vi "afd2matrix.vi"(0 "afd":cluster{i16[], i32[]}[](array[cluster])) -> (2 "Offset":dbl, 3 "Multiplier":dbl, 4 "Array":sgl[][](array[numeric]))   [LabVIEW 2010]
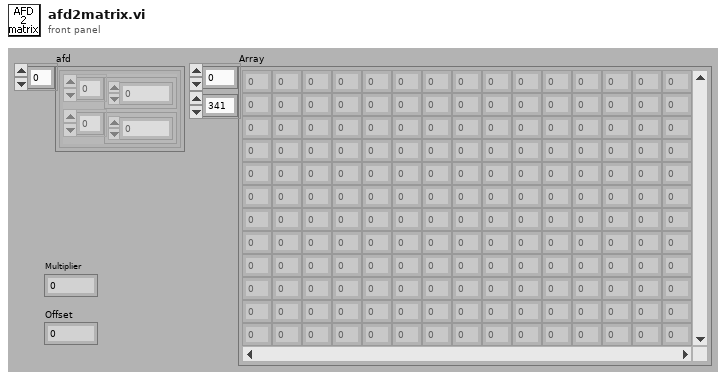
[diagram p1: front panel]
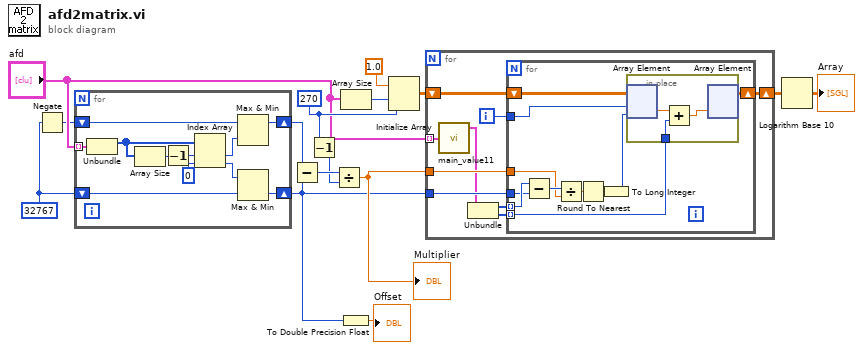
[diagram p0: block diagram]
diagram:
  w3 = i16 32767
  w8 = 270 ("dimension size")
  n1 = Negate(x=w3) -> (-x=w4:i16)
  n2 = for {
    tunnel: "afd" -> [w26] mode=indexing
    shift-right: [w17] -> w1
    shift-left: w3 -> [w16]
    shift-right: [w18] -> w2
    shift-left: w4 -> [w19]
    n3 = Unbundle(w26) -> (w22:i16[])  [unwired: 1 out]
    n4 = Array Size(array=w22) -> (size(s)=w24:i32)
    n5 = Decrement(x=w24) -> (x-1=w23:i32)
    n6 = Index Array(array=w22, index #1=w23, index #2=0 ("index")) -> (element #1=w20:i16, element #2=w21:i16)
    n7 = Max & Min(x=w19, y=w20) -> (max(x,y)=w18:i16)  [unwired: 1 out]
    n8 = Max & Min(x=w21, y=w16) -> (min(x,y)=w17:i16)  [unwired: 1 out]
  }
  n9 = Subtract(x=w2, y=w1) -> (x-y=w7:i16)
  n10 = Decrement(x=w8) -> (x-1=w6:i32)
  n11 = Divide(x=w7, y=w6) -> (x/y=w14:dbl)
  "Multiplier" <- w14
  n12 = Array Size(array="afd") -> (size(s)=w15:i32)
  n13 = To Double Precision Float(number=w1) -> (double precision float=→"Offset":dbl)
  n14 = Initialize Array(sgl 1.0 ("index"), w15, w8) -> (w13:sgl[][])
  n15 = for {
    tunnel: "afd" -> [w27] mode=indexing
    shift-right: [w34] -> w10
    shift-left: w13 -> [w35]
    tunnel: w1 -> [w32]
    tunnel: w14 -> [w31]
    i -> [w33]
    n16 = call "main_value11.vi"("hist"=w27) -> ("hist w/o main"=w30:cluster{"values":i16[], "q":i32[]})  [unwired: 3 in, 1 out]
    n17 = Unbundle(w30) -> ("values"=w29:i16[], "q"=w28:i32[])
    n18 = for {
      tunnel: w29 -> [w43] mode=indexing
      tunnel: w28 -> [w44] mode=indexing
      tunnel: w33 -> [w37]
      tunnel: w32 -> [w42]
      tunnel: w31 -> [w39]
      shift-right: [w45] -> w34
      shift-left: w35 -> [w46]
      n19 = Subtract(x=w43, y=w42) -> (x-y=w41:i16)
      n20 = Divide(x=w41, y=w39) -> (x/y=w40:dbl)
      n21 = Round To Nearest(number=w40) -> (nearest integer value=w38:dbl)
      n22 = To Long Integer(number=w38) -> (32bit integer=w36:i32)
      n23 = in-place {
        in-place-border: w44 -> [w47]
        n24 = in-place-array #1(w46, w37, w36) -> (w49:sgl)
        n25 = Add(x=w49, y=w47) -> (x+y=w48:sgl)
        n26 = in-place-array #1(w48) -> (w45:sgl[][])  [unwired: 2 out]
      }
    }
  }
  n27 = Logarithm Base 10(1:w10) -> (0:→"Array":sgl[][])
